vi "TemperatureLogging.vi"() -> ()   [LabVIEW 2019]
uses:
  C:/Program Files (x86)/National Instruments/LabVIEW 2019/examples/Instrument IO/Serial/support/Serial - Settings.ctl
  <vilib>/Instr/_visa.llb/VISA Configure Serial Port (Instr).vi
panel:
  in  "VISA resource name":refnum<visa-resource-name>="COM1"
  in  "Stop":bool
  out "Thermometer":dbl(slide) scale=0.0..100.0
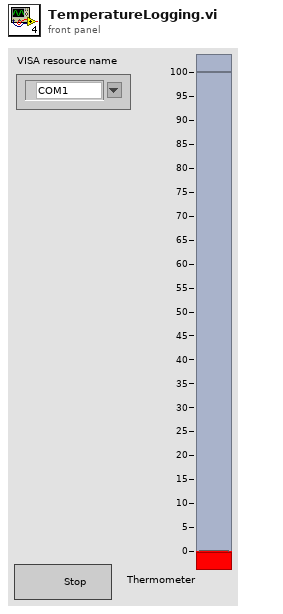
[diagram p1: front panel]
types:
  T1 = typedef "Serial - Settings.ctl" = cluster{"baud rate":u32, "data bits":u16, "parity":enum16{"None", "Odd", "Even", "Mark", "Space"}, "stop bits":u16, "flow control":u16}
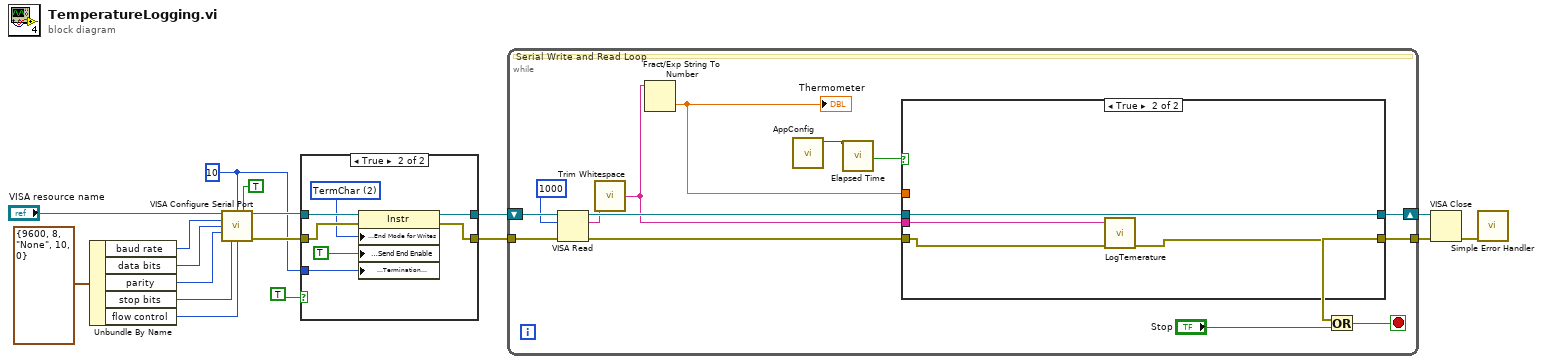
[diagram p0: block diagram]
diagram:
  w1 = u8 10 ("Termination Character")
  n1 = Unbundle By Name(T1 {"baud rate"=9600, "data bits"=8, "parity"=enum."None", "stop bits"=10, "flow control"=0} ("Serial Settings")) -> ("baud rate"=w13:u32, "data bits"=w14:u16, "parity"=w15:enum16{"None", "Odd", "Even", "Mark", "Space"}, "stop bits"=w16:u16, "flow control"=w7:u16)
  n2 = call-poly "VISA Configure Serial Port"("VISA resource name"="VISA resource name", "termination char\n(0xA = '\\n' = LF)"=w1, "Enable Termination\nChar (T)"=TRUE ("End Read on Termination Character?"), "baud rate (9600)"=w13, "data bits (8)"=w14, "parity (0:none)"=w15, "stop bits (10: 1 bit)"=w16, "flow control (0:none)"=w7) -> ("VISA resource name out"=w4:refnum<visa-resource-name>, "error out"=w6:errorcluster)  [unwired: 2 in, 4 out]
  n3 = case shown="True" TRUE ("End Write on Termination Character?") {
    tunnel: w4 -> [w18 w26]
    tunnel: w6 -> [w19 w25]
    tunnel: [w18 w24] -> w3
    tunnel: [w19 w23] -> w5
    tunnel: w1 -> [_ w21]
    frame False {
    }
    frame True {
      w22 = u16 2 items=["None", "LastBit", "TermChar", "Break"] ("Serial Settings:Serial End Mode for Writes")
      n4 = property class="Instr"(reference=w26, error in=w25, "Serial Settings:End Mode for Writes"=w22, "Message Based Settings:Send End Enable"=TRUE, "Message Based Settings:Termination Character"=w21) -> (reference out=w24:refnum<visa-resource-name>, error out=w23:errorcluster)
    }
  }
  n5 = while {
    shift-right: [w30] -> w8
    shift-left: w3 -> [w40]
    tunnel: w5 -> [w39]
    tunnel: [w33] -> w9
    stop <- w38 stop-if-true
    # "Serial Write and Read Loop"
    n6 = VISA Read(VISA resource name=w40, byte count=u32 1000 ("Read Count"), error in (no error)=w39) -> (VISA resource name out=w31:refnum<visa-resource-name>, read buffer=w29:string, error out=w34:errorcluster)  [unwired: 1 out]
    n7 = call <vilib>:"Trim Whitespace.vi"("string"=w29) -> ("trimmed string"=w28:string)  [unwired: 1 in]
    n8 = Fract/Exp String To Number(string=w28) -> (number=w35:dbl)  [unwired: 3 in, 1 out]
    "Thermometer" <- w35
    n9 = call "AppConfig.vi"() -> ("value"=w27:u32)  [unwired: 10 in, 1 out]
    n10 = call "Elapsed Time"("Time Target (s)"=w27) -> ("Time has Elapsed"=w32:bool)  [unwired: 11 in, 7 out]
    n11 = case shown="True" w32 {
      tunnel: w35 -> [_ _]
      tunnel: w34 -> [w42 w45]
      tunnel: [w42 w44] -> w33
      tunnel: w31 -> [w41 w46]
      tunnel: [w41 w46] -> w30
      tunnel: w28 -> [_ w43]
      frame False {
      }
      frame True {
        n12 = call "LogTemerature.vi"("error in (no error)"=w45, "Temp_Data"=w43) -> ("error out"=w44:errorcluster)  [unwired: 9 in]
      }
    }
    n13 = Or(x=w33, y="Stop") -> (x .or. y?=w38:bool)
  }
  n14 = VISA Close(VISA resource name=w8, error in (no error)=w9) -> (error out=w10:errorcluster)
  n15 = call <vilib>:"Simple Error Handler.vi"("error in (no error)"=w10) -> ()  [unwired: 1 in, 8 out]
